vi "CropTIFF.vi"() -> ()   [LabVIEW 2011]
uses:
  Library/tiff/TiffModules/AddTiffPage_U16_text_res.vi
panel:
  in  "hflip":bool
  in  "Clear string":bool=TRUE
  in  "Output type":u16(ring)=257 items=["Big-Endian"=0, "Native"=1, "Little-Endian"=2, "BigTiff-Big-Endian"=256, "Bigtiff,Native"=257, "Biftiff,Littleendian"=258]
  in  "Inputfile":path=path "C:/temp/20240508-Beads/I39/I39_B1_Raw.tif"
  in  "Stop at offset:":u64=429496729500
  out "AfterDIRoffset":u64 format="%09d"
  in  "y-length":i32=3691
  in  "y-start":i32=17
  in  "x-length":i32=5544
  in  "x-start":i32=86
  out "Input-page":i32
  out "string":string
  out "xy-resolution":cluster{"x":dbl, "y":dbl}
  out "Out":u16[][](graph)
  out "In":u16[][](graph)
  # "select all tiff files\nenter crop data (wie IJ!)\nrun\nnew name with _crop.tif\nstops at max tiff-offset 2^32"
  # "4294967295 for std Tiff"
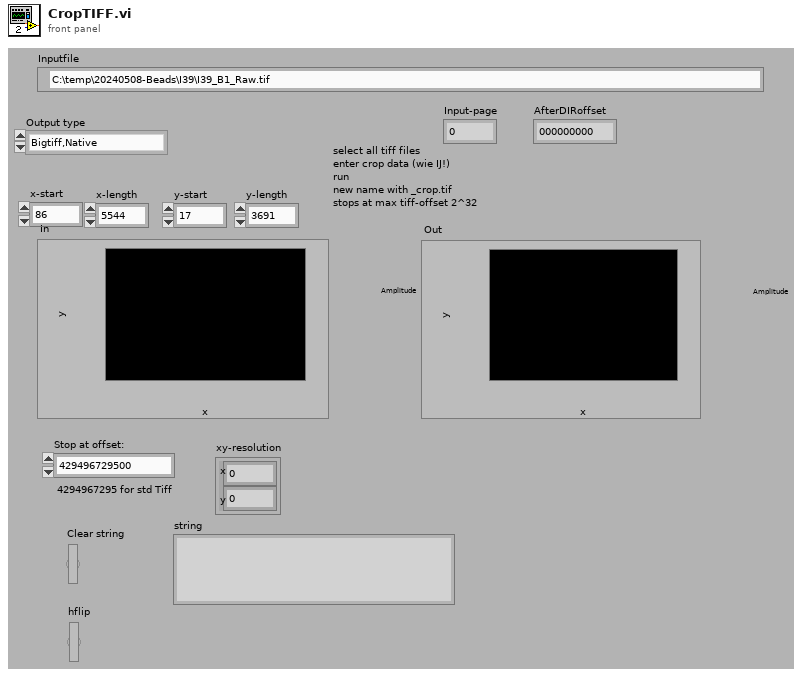
[diagram p1: front panel]
types:
  T1 = cluster{"Tiff refnum":refnum<file>, "BigTiff,Endian":u16}
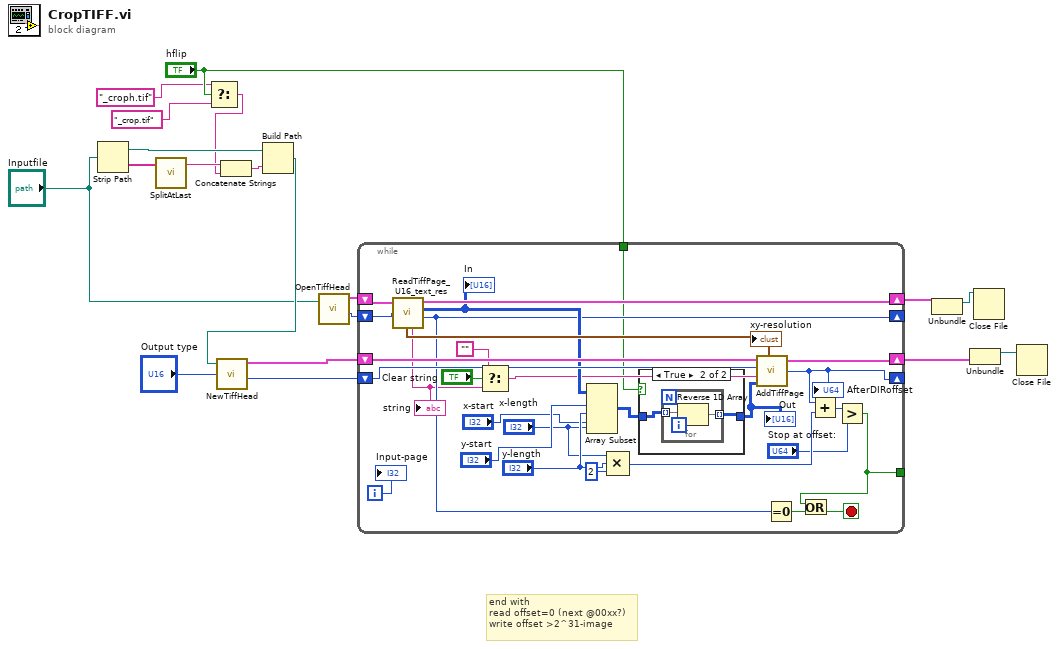
[diagram p0: block diagram]
diagram:
  # "end with \nread offset=0 (next @00xx?)\nwrite offset >2^31-image"
  n1 = Strip Path(path="Inputfile") -> (stripped path=w11:path, name=w12:string)
  n2 = call "SplitAtLast.vi"("In-String"=w12) -> ("Front (default)"=w13:string)  [unwired: 1 in, 1 out]
  n3 = Select(t="_croph.tif" ("String"), s="hflip", f="_crop.tif" ("String")) -> (s? t:f=w1:string)
  n4 = Concatenate Strings(w13, w1) -> (w19:string)
  n5 = Build Path(base path=w11, name or relative path=w19) -> (appended path=w18:path)
  n6 = call "NewTiffHead.vi"("file path"=w18, "BigTiff,Endian"="Output type") -> ("TIFF file"=w17:T1, "Place for first IFD (8,eof-position)"=w16:u64)  [unwired: 2 in, 1 out]
  n7 = call "OpenTiffHead.vi"("file path"="Inputfile") -> ("TIFF file"=w10:T1, "first Diroffset"=w9:u64)  [unwired: 2 in, 1 out]
  n8 = while {
    shift-right: [w40] -> w8
    shift-left: w10 -> [w43]
    shift-right: [w47] -> w15
    shift-left: w17 -> [w48]
    shift-right: [w38] -> _
    shift-left: w9 -> [w42]
    shift-right: [w33] -> _
    shift-left: w16 -> [w46]
    tunnel: [w28] -> _
    tunnel: "hflip" -> [w20]
    i -> [w44]
    stop <- w29 stop-if-true
    n9 = call "ReadTiffPage_U16_text_res.vi"("TIFF file"=w43, "IFDoffset"=w42) -> ("Pixelsize [µm]"=w41:cluster{"x":dbl, "y":dbl}, "TIFF file out"=w40:T1, "16-bit pixmap"=w39:u16[][], "string"=w25:string, "Next offset"=w38:i64)  [unwired: 3 in, 1 out]
    "In" <- w39
    "xy-resolution" <- w41
    "string" <- w25
    n10 = Select(t="", s="Clear string", f=w25) -> (s? t:f=w26:string)
    n11 = Array Subset(array=w39, index (row)="y-start", length (row)="y-length", index (col)="x-start", length (col)="x-length") -> (w22:u16[][])
    n12 = Compound Arithmetic op=MULTIPLY("x-length", "y-length", 2 ("value")) -> (w32:i32)
    n13 = case shown="True" w20 {
      tunnel: w22 -> [w49 w51]
      tunnel: [w49 w50] -> w21
      frame False {
      }
      frame True {
        n14 = for {
          tunnel: w51 -> [w53] mode=indexing
          tunnel: [w52] -> w50 mode=indexing
          n15 = Reverse 1D Array(array=w53) -> (reversed array=w52:u16[])
        }
      }
    }
    "Out" <- w21
    n16 = call-poly "AddTiffPage.vi"("TIFF file"=w48, "After last DIROffset"=w46, "Text"=w26, "16-bit pixmap x, y"=w21, "Pixelsize [µm]"=w41) -> ("TIFF file"=w47:T1, "AfterDIRoffset"=w33:u64)  [unwired: 1 out]
    "AfterDIRoffset" <- w33
    n17 = Equal To 0?(x=w38) -> (x = 0?=w45:bool)
    n18 = Add(x=w33, y=w32) -> (x+y=w31:u64)
    n19 = Greater?(x=w31, y="Stop at offset:") -> (0:w28:bool)
    n20 = Or(x=w28, y=w45) -> (x .or. y?=w29:bool)
    "Input-page" <- w44
  }
  n21 = Unbundle(w8) -> ("Tiff refnum"=w7:refnum<file>)  [unwired: 1 out]
  n22 = Unbundle(w15) -> ("Tiff refnum"=w14:refnum<file>)  [unwired: 1 out]
  n23 = Close File(refnum=w7) -> ()  [unwired: 1 in, 2 out]
  n24 = Close File(refnum=w14) -> ()  [unwired: 1 in, 2 out]
